vi "GV_GetControlRef.vi"(8 "error in (no error)":errorcluster, 9 "CNT name":string, 11 "Gviewer in":refnum<class "Gviewer.lvclass">) -> (0 "error out":errorcluster, 1 "Reference":refnum<vi>, 3 "Gviewer out":refnum<class "Gviewer.lvclass">)   [LabVIEW 2020, in "Sgraph_lib_V1.lvlib" / "Gviewer.lvclass"]
doc: "Get the reference of a FrontPanel control"
uses:
  Gviewer.lvclass
  Gviewer.lvclass/Gviewer.ctl
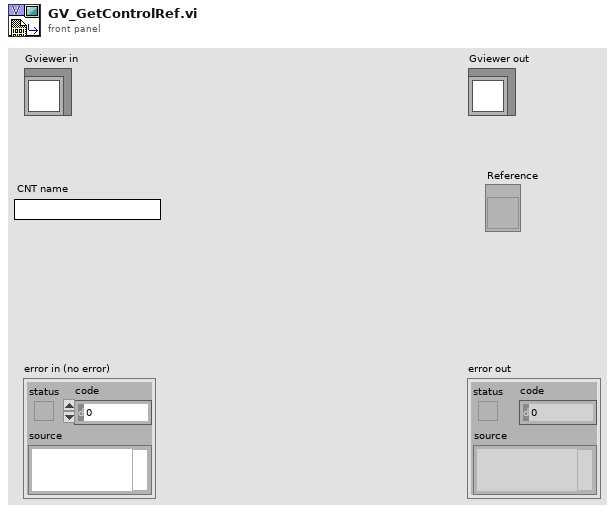
[diagram p1: front panel]
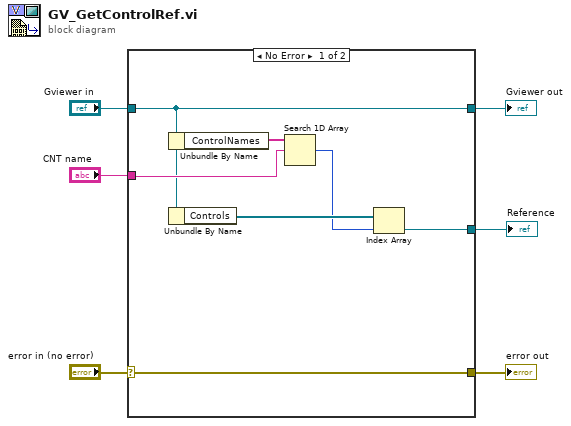
[diagram p0: block diagram]
diagram:
  n1 = case shown="No Error" "error in (no error)" {
    selector: "error in (no error)" -> [w13 w15]
    tunnel: [w13 w15] -> w5
    tunnel: [w10 w14] -> w3
    tunnel: "Gviewer in" -> [w10 w14]
    tunnel: "CNT name" -> [w11 _]
    tunnel: [w7 _] -> w1
    frame No Error {
      n2 = Unbundle By Name(w10) -> ("ControlNames"=w12:string[])
      n3 = Unbundle By Name(w10) -> ("Controls"=w9:refnum<vi>[])
      n4 = Search 1D Array(1D array=w12, element=w11) -> (index of element=w8:i32)  [unwired: 1 in]
      n5 = Index Array(array=w9, index=w8) -> (element=w7:refnum<vi>)
    }
    frame Error {
    }
  }
  "error out" <- w5
  "Gviewer out" <- w3
  "Reference" <- w1
